vi "CST_1299MainShifter.vi"() -> (1 "Main Shifter":T1 {"Vref" format="%.03pV"; "f(CLK)" format="%.04pHz"; "RegMap Data"."Base" format="%.0x"; "RegMap Data"."Item Count" format="%.0x"; "RegMap Data"."Value" format="%.0x"; "RegMap Data"."RegMap"."Mask" format="%.0x"; "RegMap Data"."Default" format="%.0x"; "RegMap Data"."Register" format="%.0x"})   [LabVIEW 2010]
uses:
  Controls/Shift Registers/TYP_1299MainShifter.ctl
  Modules/Scan RegMap/TYP_ADSxxxx Register.ctl
  Modules/Scan RegMap/TYP_RegMap Item.ctl
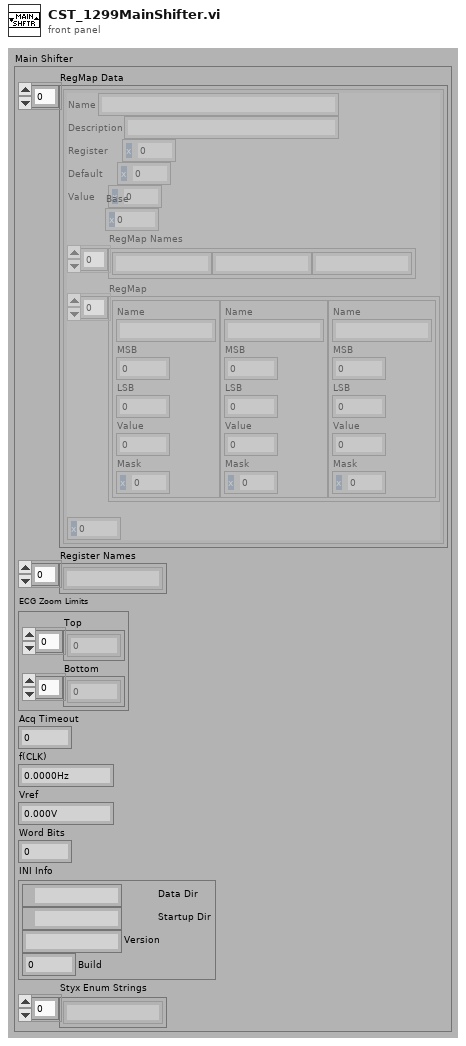
[diagram p1: front panel]
types:
  T1 = typedef "TYP_1299MainShifter.ctl" = cluster{"RegMap Data":T2[], "Register Names":string[], "ECG Zoom Limits":cluster{"Top":i32[], "Bottom":i32[]}, "Acq Timeout":u16, "f(CLK)":dbl, "Vref":dbl, "Word Bits":i32, "INI Info":cluster{"Data Dir":path, "Startup Dir":path, "Version":string, "Build":i16}, "Styx Enum Strings":string[]}
  T2 = typedef "TYP_ADSxxxx Register.ctl" = cluster{"Name":string, "Description":string, "Register":u16, "Default":u16, "Value":u16, "Base":u16, "RegMap Names":string[], "RegMap":T3[], "Item Count":u8}
  T3 = typedef "TYP_RegMap Item.ctl" = cluster{"Name":string, "MSB":u16, "LSB":u16, "Value":u16, "Mask":u16}
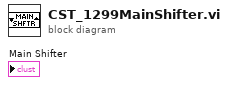
[diagram p0: block diagram]
diagram:
